vi "PM9_TCP_READ-SN.vi"(0 "VISA":refnum<visa-resource-name>="TCPIP0::169.254.70.190::502::SOCKET", 5 "connection ID":refnum<k5>, 11 "error in (no error)":errorcluster, 14 "Close tcp(t)":bool) -> (2 "Dev OK(t)":bool, 3 "SN":string, 4 "visa out":refnum<visa-resource-name>, 6 "connection ID out":refnum<k5>, 8 "Model":string, 13 "Device Info":string, 15 "error out":errorcluster)   [LabVIEW 2018]
panel:
  out "data out 2":string
  # "Use a valid connection id to run in loop"
  # "MFR"
  # "MODEL"
  # "S/N"
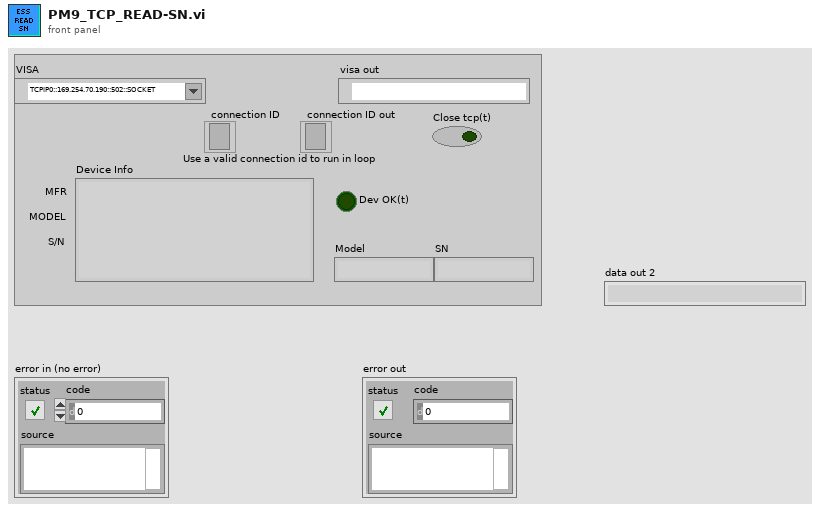
[diagram p1: front panel]
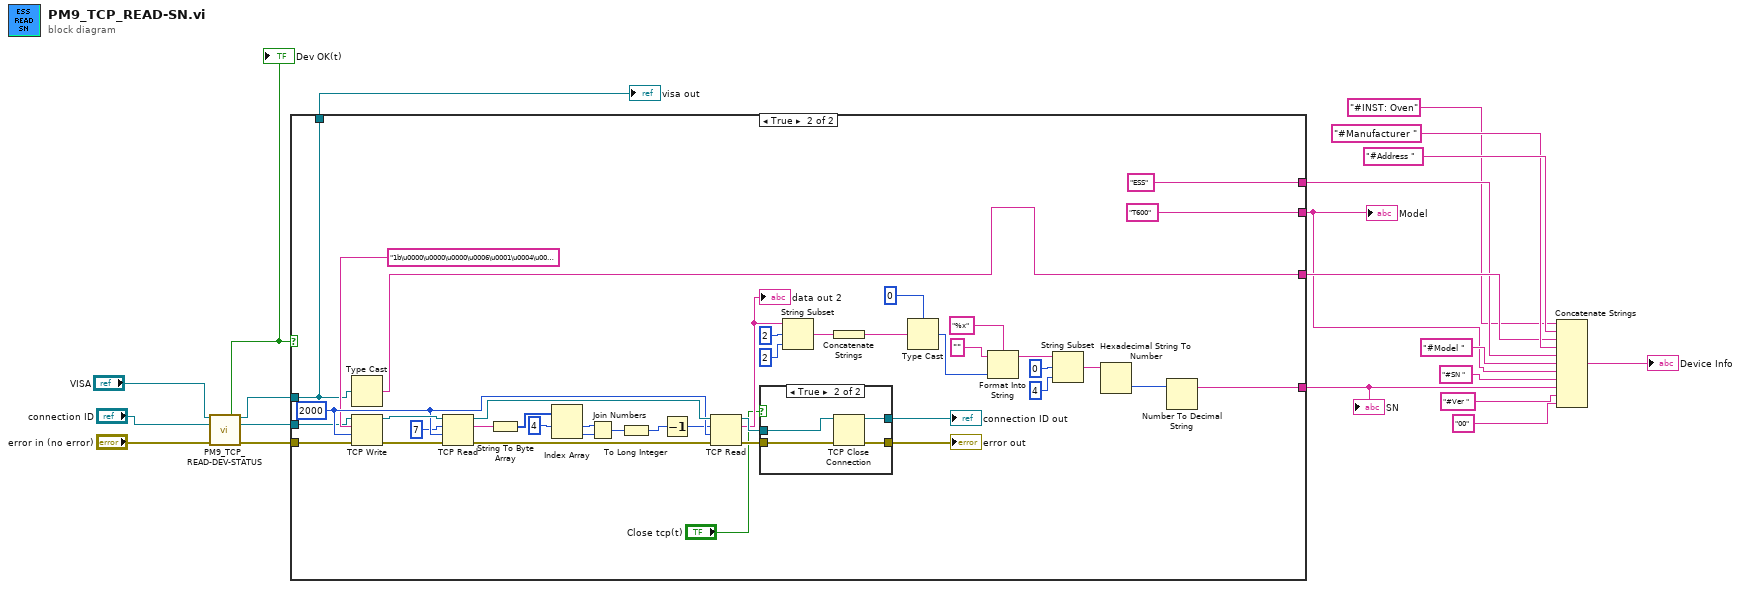
[diagram p0: block diagram]
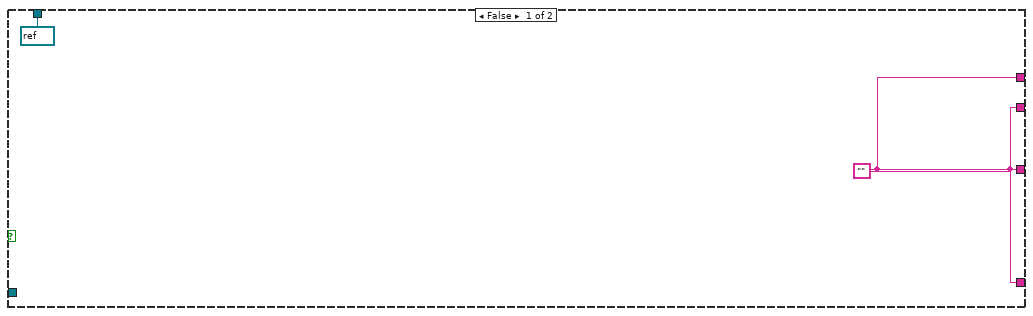
[diagram p2: hidden frame]
diagram:
  n1 = call "PM9_TCP_READ-DEV-STATUS.vi"("VISA"="VISA", "connection ID"="connection ID", "error in (no error)"="error in (no error)") -> ("Dev OK(t)"=w5:bool, "visa out"=w4:refnum<visa-resource-name>, "connection ID out"=w6:refnum<k5>, "error out"=w7:errorcluster)  [unwired: 9 in]
  "Dev OK(t)" <- w5
  n2 = case shown="True" w5 {
    tunnel: [w22 w23] -> w15
    tunnel: [w22 w29] -> w14
    tunnel: [w22 "ESS" ("string")] -> w12
    tunnel: [w22 "T600" ("string")] -> w11
    tunnel: w4 -> [_ w24]
    tunnel: w7 -> [_ w26]
    tunnel: w6 -> [_ w25]
    tunnel: [refnum<visa-resource-name> refnum ("visa out") w24] -> w3
    frame False {
      w22 = ""
    }
    frame True {
      w57 = 2000 ("timeout ms (25000)")
      n3 = Type Cast(x=w24) -> (*(type *) &x=w23:string)  [unwired: 1 in]
      n4 = TCP Write(connection ID=w25, data in="1b\u0000\u0000\u0000\u0006\u0001\u0004\u0000\f\u0000\u0002" ("address"), error in (no error)=w26, 9:w57) -> (connection ID out=w61:refnum<k5>, error out=w59:errorcluster)  [unwired: 1 out]
      n5 = TCP Read(connection ID=w61, bytes to read=7, error in (no error)=w59, 9:w57) -> (connection ID out=w60:refnum<k5>, data out=w49:string, error out=w58:errorcluster)  [unwired: 1 in]
      n6 = String To Byte Array(string=w49) -> (unsigned byte array=w50:u8[])
      n7 = Index Array(array=w50, index #1=4 ("index")) -> (element #1=w51:u8, element #2=w52:u8)  [unwired: 1 in]
      n8 = Join Numbers(hi=w51, lo=w52) -> ((hi.lo)=w54:u16)
      n9 = To Long Integer(number=w54) -> (32bit integer=w53:i32)
      n10 = Decrement(x=w53) -> (x-1=w48:i32)
      n11 = TCP Read(connection ID=w60, bytes to read=w48, error in (no error)=w58, 9:w57) -> (connection ID out=w63:refnum<k5>, data out=w45:string, error out=w62:errorcluster)  [unwired: 1 in]
      "data out 2" <- w45
      n12 = case shown="True" "Close tcp(t)" {
        tunnel: w63 -> [w65 w69]
        tunnel: w62 -> [w64 w68]
        tunnel: [w64 w67] -> w31
        tunnel: [w65 w66] -> w43
        frame False {
        }
        frame True {
          n13 = TCP Close Connection(connection ID=w69, error in (no error)=w68) -> (connection ID out=w66:refnum<k5>, error out=w67:errorcluster)  [unwired: 1 in]
        }
      }
      "error out" <- w31
      "connection ID out" <- w43
      n14 = String Subset(string=w45, offset (0)=u16 2 ("bytes to read"), length (rest)=u16 2 ("bytes to read")) -> (substring=w39:string)
      n15 = Concatenate Strings(w39) -> (w40:string)
      n16 = Type Cast(type=0, x=w40) -> (*(type *) &x=w38:i32)
      n17 = Format Into String(format string="%x", initial string="", w38) -> (resulting string=w35:string)  [unwired: 1 in, 1 out]
      n18 = String Subset(string=w35, offset (0)=0, length (rest)=4 ("length (rest)")) -> (substring=w32:string)
      n19 = Hexadecimal String To Number(string=w32) -> (number=w30:u32)  [unwired: 2 in, 1 out]
      n20 = Number To Decimal String(number=w30) -> (decimal integer string=w29:string)  [unwired: 1 in]
    }
  }
  "Model" <- w11
  "visa out" <- w3
  "SN" <- w14
  n21 = Concatenate Strings("#INST: Oven" ("string"), "#Address " ("string"), w15, "#Manufacturer ", w12, "#Model ", w11, "#SN " ("string"), w14, "#Ver " ("string"), "00" ("string")) -> (→"Device Info":string)
